vi "CreatePrivateEvents.vi"(8 "error in (no error)":errorcluster, 11 "Measurement.Free":refnum<class "Measurement.Free.lvclass">) -> (0 "error out":errorcluster, 3 "Measurement.Free out":refnum<class "Measurement.Free.lvclass">)   [LabVIEW 2017, in "Measurement.Free.lvclass"]
doc: "JKI State Machine Objects (SMO) 1.1.0.20\nJKI - JKI\nCopyright (c) 2016, JKI"
uses:
  Measurement.Free.lvclass
  Measurement.Free.lvclass/Measurement.Free.ctl
  Typedefs/PrivateEvents--Measurement.Free.Initialize.ctl
  <vilib>/JKI/JKI SMO/SMO/SMO.lvclass
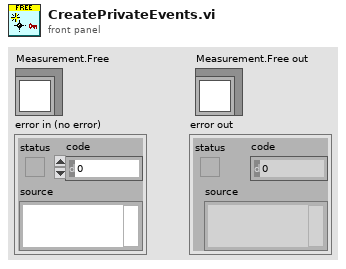
[diagram p1: front panel]
types:
  T1 = typedef "Measurement.Free.lvclass/PrivateData--Ref.ctl" = refnum<data-value>
  T2 = typedef "Measurement.Free.lvclass/PrivateEvents--Measurement.Free.Initialize.ctl" = bool
  T3 = typedef "Measurement.Free.lvclass/PrivateData--Cluster.ctl" = cluster{"Configuration":T4, "Public Events":T14, "Protected Events":T15, "Private Events":T16, "Data":T17}
  T4 = typedef "Measurement.Free.lvclass/Configuration--Cluster.ctl" = cluster{"Measurement.Type":enum16{"Free", "I/V Curve", "Wavelength sweeping", "Photocurrent mapping"}, "Configuration.Hardware":T5}
  T5 = typedef "Measurement.Free.lvclass/Configuration.Hardware--Cluster.ctl" = cluster{"Configuration.SMU":T6, "Configuration.LIA":T8, "Configuration.OPM":T10, "Configuration.OPA":T12}
  T6 = typedef "Measurement.Free.lvclass/Configuration.SMU--Cluster.ctl" = cluster{"SMU Model":string, "Configuration":T7}
  T7 = typedef "SMU.lvclass/Configuration--Cluster.ctl" = cluster{"VISA Resource":string, "Channel":string}
  T8 = typedef "Measurement.Free.lvclass/Configuration.LIA--Cluster.ctl" = cluster{"LIA Model":string, "Configuration":T9}
  T9 = typedef "LIA.lvclass/Configuration--Cluster.ctl" = cluster{"VISA Resource":string}
  T10 = typedef "Measurement.Free.lvclass/Configuration.OPM--Cluster.ctl" = cluster{"OPM Model":string, "Configuration":T11}
  T11 = typedef "OPM.lvclass/Configuration--Cluster.ctl" = cluster{"VISA Resource":string}
  T12 = typedef "Measurement.Free.lvclass/Configuration.OPA--Cluster.ctl" = cluster{"OPA Model":string, "Configuration":T13}
  T13 = typedef "OPA.lvclass/Configuration--Cluster.ctl" = cluster{"Serial Number":string}
  T14 = typedef "Measurement.Free.lvclass/PublicEvents--Cluster.ctl" = cluster{"Data Changed":refnum<user-event>}
  T15 = typedef "Measurement.Free.lvclass/ProtectedEvents--Cluster.ctl" = cluster{"API_Template":refnum<user-event>}
  T16 = typedef "Measurement.Free.lvclass/PrivateEvents--Cluster.ctl" = cluster{"Initialize":refnum<user-event>}
  T17 = typedef "Measurement.Free.lvclass/Data.ctl" = string
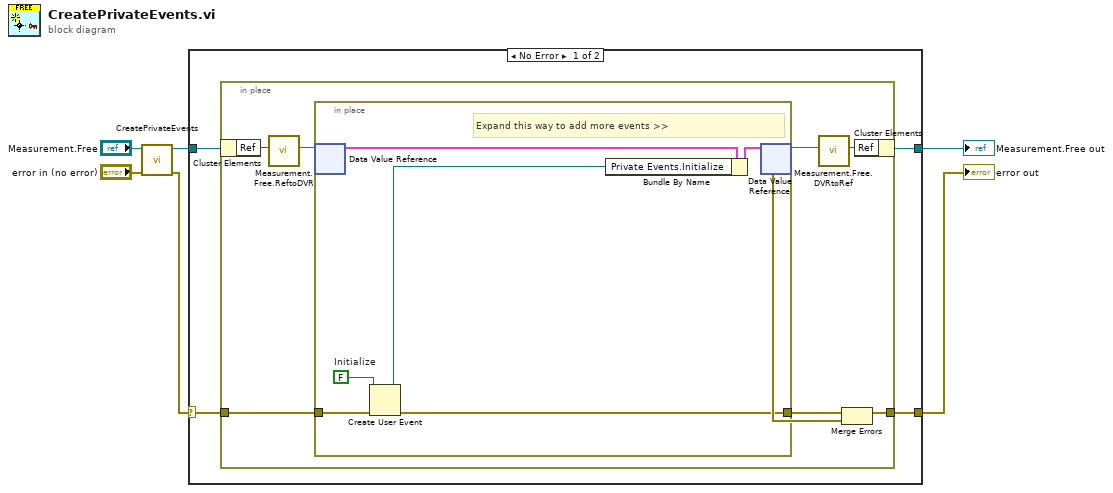
[diagram p0: block diagram]
diagram:
  n1 = call-parent "CreatePrivateEvents.vi"("error in (no error)"="error in (no error)", "SMO"="Measurement.Free") -> ("error out"=w4:errorcluster, "SMO out"=w2:refnum<class "Measurement.Free.lvclass">)  [unwired: 8 in]
  n2 = case shown="No Error" w4 {
    selector: w4 -> [w8 w26]
    tunnel: [w7 w26] -> w3
    tunnel: [w9 w25] -> w1
    tunnel: w2 -> [w10 w25]
    frame No Error {
      n3 = in-place {
        in-place-border: w8 -> [w18]
        in-place-border: [w15] -> w7
        n4 = in-place-cluster #1(w10) -> ("Ref"=w14:u32)
        n5 = call "Measurement.Free.ReftoDVR.vi"("Ref"=w14) -> ("Ref"=w13:T1)  [unwired: 10 in]
        n6 = in-place {
          in-place-border: w18 -> [w23]
          in-place-border: [w21] -> w17
          w20 = T2 FALSE  # Initialize
          # "Expand this way to add more events >>"
          n7 = in-place-dvr #2(w13) -> (w22:T3)  [unwired: 1 out]
          n8 = Create User Event(user event datatype=w20, error in=w23) -> (user event=w19:refnum<user-event>, error out=w21:errorcluster)
          n9 = Bundle By Name(cluster=w22, "Private Events.Initialize"=w19) -> (w24:T3)
          n10 = in-place-dvr #2(w24) -> (w12:T1, w16:errorcluster)
        }
        n11 = call "Measurement.Free.DVRtoRef.vi"("Ref"=w12) -> ("Ref"=w11:u32)  [unwired: 10 in]
        n12 = Merge Errors(w17, w16) -> (w15:errorcluster)
        n13 = in-place-cluster #1("Ref"=w11) -> (w9:refnum<class "Measurement.Free.lvclass">)
      }
    }
    frame Error {
    }
  }
  "error out" <- w3
  "Measurement.Free out" <- w1
